vi "Does Rect Contains Point.vi"(9 "point":cluster{"x":i16, "y":i16}, 11 "rect":T1) -> (2 "Contained?":bool)   [LabVIEW 2015]
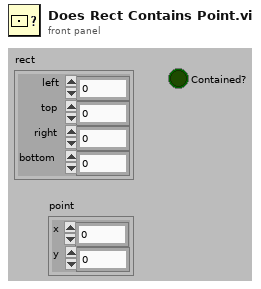
[diagram p1: front panel]
types:
  T1 = cluster{"left":i16, "top":i16, "right":i16, "bottom":i16}
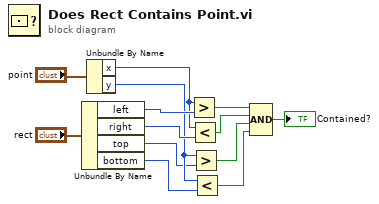
[diagram p0: block diagram]
diagram:
  n1 = Unbundle By Name("rect") -> ("left"=w11:i16, "right"=w9:i16, "top"=w7:i16, "bottom"=w6:i16)
  n2 = Unbundle By Name("point") -> ("x"=w10:i16, "y"=w8:i16)
  n3 = Greater?(x=w10, y=w11) -> (0:w5:bool)
  n4 = Less?(x=w10, y=w9) -> (x < y?=w4:bool)
  n5 = Greater?(x=w8, y=w7) -> (0:w3:bool)
  n6 = Less?(x=w8, y=w6) -> (x < y?=w2:bool)
  n7 = Compound Arithmetic op=AND(w5, w4, w3, w2) -> (→"Contained?":bool)
